vi "Rename items.vi"(10 "New Name":string="NewName", 11 "Pattern":string="Template") -> ()   [LabVIEW 2019, in "ProjectItem.lvclass"]
uses:
  ProjectItem.lvclass
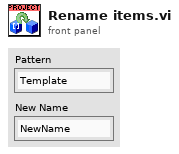
[diagram p1: front panel]
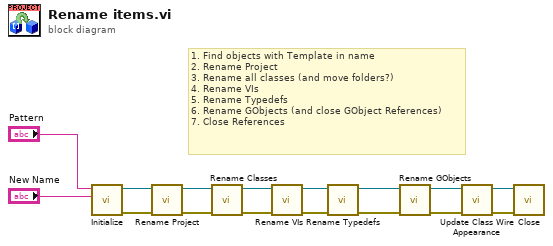
[diagram p0: block diagram]
diagram:
  # "1. Find objects with Template in name\n2. Rename Project\n3. Rename all classes (and move folders?)\n4. Rename VIs\n5. Rename Typedefs\n6. Rename GObjects (and close GObject References)\n7. Close References"
  n1 = call "Initialize.vi"("New Name"="New Name", "Pattern"="Pattern") -> ("error out"=w16:errorcluster, "ProjectItem out"=w15:refnum<class "ProjectItem.lvclass">)  [unwired: 8 in]
  n2 = call "Rename Project.vi"("error in (no error)"=w16, "ProjectItem in"=w15) -> ("error out"=w5:errorcluster, "ProjectItem out"=w6:refnum<class "ProjectItem.lvclass">)  [unwired: 8 in]
  n3 = call "Rename Classes.vi"("error in (no error)"=w5, "ProjectItem in"=w6) -> ("error out"=w3:errorcluster, "ProjectItem out"=w4:refnum<class "ProjectItem.lvclass">)  [unwired: 8 in]
  n4 = call "Rename VIs.vi"("error in (no error)"=w3, "ProjectItem in"=w4) -> ("error out"=w2:errorcluster, "ProjectItem out"=w1:refnum<class "ProjectItem.lvclass">)  [unwired: 8 in]
  n5 = call "Rename Typedefs.vi"("error in (no error)"=w2, "ProjectItem in"=w1) -> ("error out"=w8:errorcluster, "ProjectItem out"=w7:refnum<class "ProjectItem.lvclass">)  [unwired: 8 in]
  n6 = call "Rename GObjects.vi"("error in (no error)"=w8, "ProjectItem in"=w7) -> ("error out"=w10:errorcluster, "ProjectItem out"=w12:refnum<class "ProjectItem.lvclass">)  [unwired: 8 in]
  n7 = call "Update Class Wire Appearance.vi"("error in (no error)"=w10, "ProjectItem in"=w12) -> ("error out"=w9:errorcluster, "ProjectItem out"=w11:refnum<class "ProjectItem.lvclass">)  [unwired: 8 in]
  n8 = call "Close.vi"("error in (no error)"=w9, "ProjectItem in"=w11) -> ()  [unwired: 8 in, 2 out]
